vi "Read Transceiver Response.vi"(8 "error in (no error)":errorcluster, 9 "timeout in ms (0)":i32, 11 "Transceiver Interface in":refnum<class "Transceiver Interface.lvclass">) -> (0 "error out":errorcluster, 1 "empty?":bool, 2 "response":T1, 3 "Transceiver Interface out":refnum<class "Transceiver Interface.lvclass">, 4 "# elements":u32)   [LabVIEW 2017, in "Data Sharing Framework Engine.lvlib" / "Transceiver Interface.lvclass"]
uses:
  Transceiver Interface.lvclass
  C:/github/data-sharing-framework/Source/Data Sharing Framework Core/Engine/Interfaces/Engine Interface/Engine Interface.lvclass
  Response Data.ctl
  Response.ctl
  Response Parameters.ctl
  Engine Interface/Engine Interface.lvclass/Engine Interface.ctl
  Debug/Debug Flags FIFO/Debug Flags FIFO.lvclass/Debug Flags FIFO.ctl
  Engine Interface/Get Debug Flags.vi
  Engine Interface/Read 16B RT FIFO.vi
  Engine Interface/Get Response FIFO.vi
  Debug/Debug Flags FIFO/Get Infinite Timeouts.vi
  Engine Interface/Engine Interface.lvclass
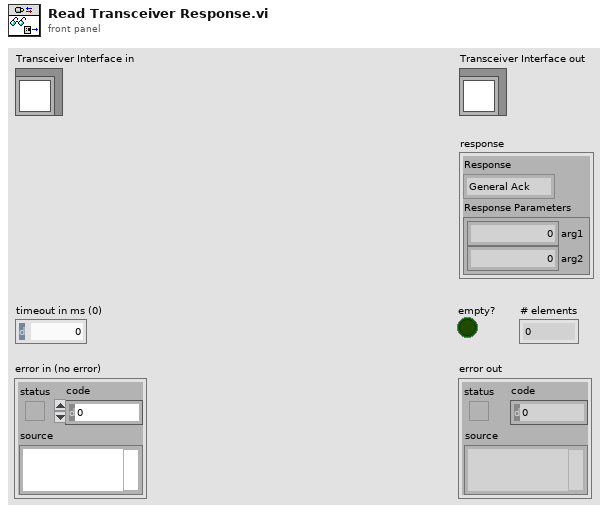
[diagram p1: front panel]
types:
  T1 = typedef "Data Sharing Framework Engine.lvlib/Transceiver Interface.lvclass/Response Data.ctl" = cluster{"Response":T2, "Response Parameters":T3}
  T2 = typedef "Data Sharing Framework Engine.lvlib/Transceiver Interface.lvclass/Response.ctl" = enum8{"General Ack", "Shutting Down"}
  T3 = typedef "Data Sharing Framework Engine.lvlib/Transceiver Interface.lvclass/Response Parameters.ctl" = cluster{"arg1":u64, "arg2":u64}
  T4 = typedef "Data Sharing Framework Engine.lvlib/Engine Interface.lvclass/16B Data.ctl" = cluster{"Command":u8, "Payload":T5}
  T5 = typedef "Data Sharing Framework Engine.lvlib/Engine Interface.lvclass/16B Payload.ctl" = cluster{"arg1":u64, "arg2":u64}
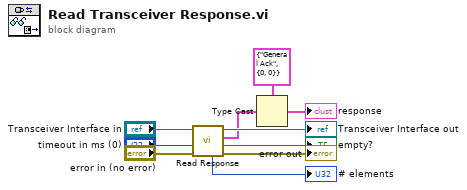
[diagram p0: block diagram]
diagram:
  n1 = call "Read Response.vi"("error in (no error)"="error in (no error)", "timeout in ms (0)"="timeout in ms (0)", "Interface in"="Transceiver Interface in") -> ("error out"=→"error out":errorcluster, "timed out?"=→"empty?":bool, "response"=w6:T4, "Interface out"=→"Transceiver Interface out":refnum<class "Transceiver Interface.lvclass">, "# elements"=→"# elements":u32)  [unwired: 4 in]
  n2 = Type Cast(type=T1 {"Response"=enum."General Ack", "Response Parameters"={"arg1"=0, "arg2"=0}} ("Plugin Response"), x=w6) -> (*(type *) &x=→"response":T1)
